vi "Select LabVIEW Version.vi"(11 "EXE Name":string) -> (2 "Exe Path Specified":bool, 3 "LabVIEW Path":path)   [LabVIEW 2018]
panel:
  in  "Version List":i32(listbox)
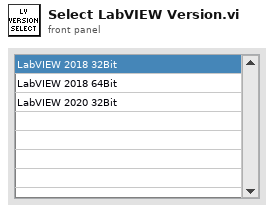
[diagram p1: front panel]
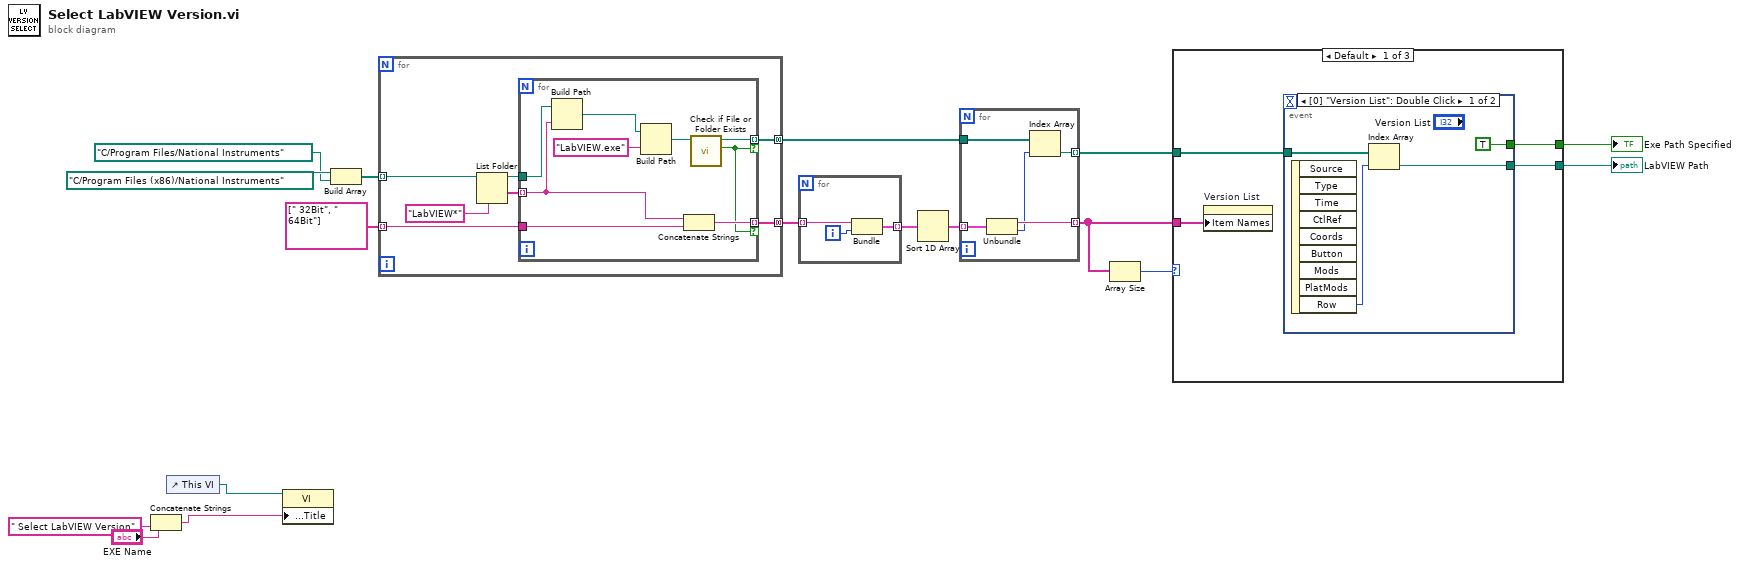
[diagram p0: block diagram]
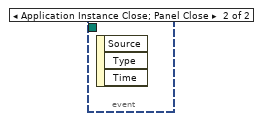
[diagram p2: hidden frame]
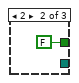
[diagram p3: hidden frame]
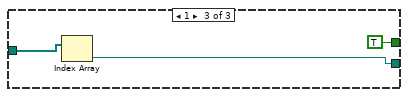
[diagram p4: hidden frame]
diagram:
  n1 = Concatenate Strings("EXE Name", " Select LabVIEW Version" ("string")) -> (w4:string)
  n2 = control-ref of="This VI"() -> (w6:refnum<vi>)
  n3 = property class="VI"(reference=w6, "Front Panel.Title"=w4) -> ()  [unwired: 1 in, 2 out]
  n4 = Build Array(path "C:/Program Files (x86)/National Instruments", path "C:/Program Files/National Instruments") -> (w15:path[])
  n5 = for {
    tunnel: w15 -> [w23] mode=indexing
    tunnel: [w21] -> w11 mode=concatenating
    tunnel: string[] [" 32Bit", " 64Bit"] -> [w20] mode=indexing
    tunnel: [w18] -> w8 mode=concatenating
    n6 = List Folder(path=w23, pattern="LabVIEW*") -> (path out=w19:path, folder names=w22:string[])  [unwired: 2 in, 2 out]
    n7 = for {
      tunnel: w22 -> [w25] mode=indexing
      tunnel: [w33] -> w21 mode=indexing if=w26
      tunnel: w20 -> [w32]
      tunnel: w19 -> [w31]
      tunnel: [w27] -> w18 mode=indexing if=w26
      n8 = Build Path(base path=w31, name or relative path=w25) -> (appended path=w30:path)
      n9 = Build Path(base path=w30, name or relative path="LabVIEW.exe") -> (appended path=w28:path)
      n10 = Concatenate Strings(w25, w32) -> (w33:string)
      n11 = call <vilib>:"Check if File or Folder Exists.vi"("path"=w28) -> ("file or folder exists?"=w26:bool, "dup path"=w27:path)  [unwired: 8 in, 1 out]
    }
  }
  n12 = for {
    tunnel: w11 -> [w35] mode=indexing
    tunnel: [w34] -> w10 mode=indexing
    i -> [w36]
    n13 = Bundle(w35, w36) -> (w34:cluster{string, i32})  [unwired: 1 in]
  }
  n14 = Sort 1D Array(array=w10) -> (sorted array=w9:cluster{string, i32}[])
  n15 = for {
    tunnel: w9 -> [w41] mode=indexing
    tunnel: [w40] -> w2 mode=indexing
    tunnel: w8 -> [w39]
    tunnel: [w37] -> w7 mode=indexing
    n16 = Unbundle(w41) -> (w40:string, w38:i32)
    n17 = Index Array(array=w39, index=w38) -> (element=w37:path)
  }
  n18 = Array Size(array=w2) -> (size(s)=w1:i32)
  n19 = case shown="Default" w1 {
    tunnel: [w45 _ w52] -> w13
    tunnel: [w44 FALSE TRUE] -> w12
    tunnel: w7 -> [w43 _ w53]
    tunnel: w2 -> [w42 _ _]
    frame Default {
      n20 = property on="Version List" class="LstBox (strict)"("Item Names"=w42) -> ()  [unwired: 2 in, 2 out]
      n21 = event shown="[0] \"Version List\": Double Click" {
        selector: _ -> [_ _]
        dyn-events: _ -> [_ _]
        timeout: _ -> [_ _]
        tunnel: w43 -> [w49 _]
        tunnel: [w48 _] -> w45
        tunnel: [TRUE _] -> w44
        event "Version List": Double Click {
          n22 = event-data() -> ("Row"=w46:i32)  [unwired: 1 in, 8 out]
          n23 = Index Array(array=w49, index=w46) -> (element=w48:path)
        }
        event Application Instance Close; Panel Close {
          n24 = event-data() -> ()  [unwired: 1 in, 3 out]
        }
      }
    }
    frame 2 {
    }
    frame 1 {
      n25 = Index Array(array=w53) -> (element=w52:path)  [unwired: 1 in]
    }
  }
  "LabVIEW Path" <- w13
  "Exe Path Specified" <- w12
